vi "IOP Calibration.vi"(11 "IOP Input [V]":dbl[](array[numeric])=[0.0, 0.0, 0.0, 0.0] caption="IOP Input") -> (3 "IOP Output [mmHg]":dbl[](array[numeric]))   [LabVIEW 2016]
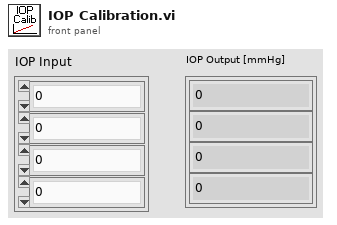
[diagram p1: front panel]
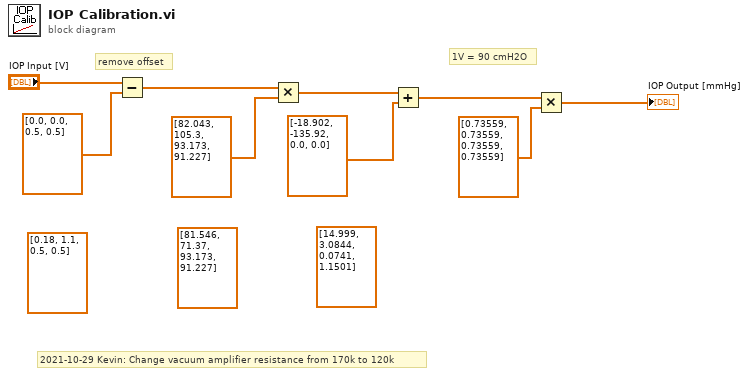
[diagram p0: block diagram]
diagram:
  (unwired) dbl[] [0.18, 1.1, 0.5, 0.5]
  (unwired) dbl[] [81.546, 71.37, 93.173, 91.227]
  (unwired) dbl[] [14.999, 3.0844, 0.0741, 1.1501]
  # "2021-10-29 Kevin: Change vacuum amplifier resistance from 170k to 120k"
  # "remove offset"
  # "1V = 90 cmH2O"
  n1 = Subtract(x="IOP Input [V]", y=dbl[] [0.0, 0.0, 0.5, 0.5]) -> (x-y=w7:dbl[])
  n2 = Multiply(x=w7, y=dbl[] [82.043, 105.3, 93.173, 91.227]) -> (x*y=w4:dbl[])
  n3 = Add(x=w4, y=dbl[] [-18.902, -135.92, 0.0, 0.0]) -> (x+y=w3:dbl[])
  n4 = Multiply(x=w3, y=dbl[] [0.73559, 0.73559, 0.73559, 0.73559]) -> (x*y=→"IOP Output [mmHg]":dbl[])
